vi "WPI_CounterOpen.vi"   [LabVIEW 2017]
doc: "Opens and configures a reference to the counter you specify, and then starts the counter. Use a separate Open VI for each counter you want to configure. You must open a reference before using any other VIs on the Counter VIs palette. You must manually select the polymorphic instance you want to use.\n\nThis software is licensed. Open the labview\\readme\\WPI Robotics Library Open Source License.txt file for more information."
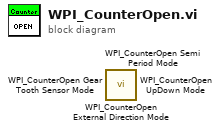
[diagram p0: block diagram]
diagram:
  n1 = call <vilib>:"WPI_CounterOpen External Direction Mode.vi"() -> ()  [unwired: 10 in, 2 out]
  n2 = call <vilib>:"WPI_CounterOpen Semi Period Mode.vi"() -> ()  [unwired: 10 in, 2 out]
  n3 = call <vilib>:"WPI_CounterOpen Gear Tooth Sensor Mode.vi"() -> ()  [unwired: 10 in, 2 out]
  n4 = call <vilib>:"WPI_CounterOpen UpDown Mode.vi"() -> ()  [unwired: 10 in, 2 out]
